vi "SetMethods.vi"(8 "error in (no error)":errorcluster, 10 "Methods":string[](array[string])=["Draw ()", "Scale ()", "Move ()"], 11 "UMLClass in":refnum<class "UMLClass.lvclass">) -> (0 "error out":errorcluster, 3 "UMLClass out":refnum<class "UMLClass.lvclass">)   [LabVIEW 2021, in "Picture2D.lvlib" / "UMLClass.lvclass"]
uses:
  UMLClass.lvclass
  UMLClass.lvclass/UMLClass.ctl
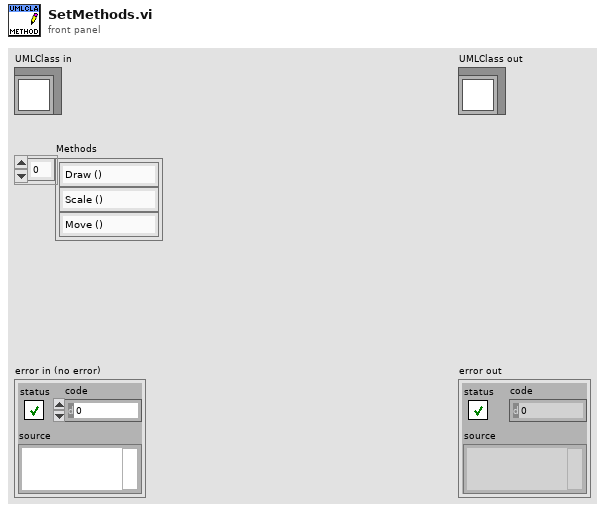
[diagram p1: front panel]
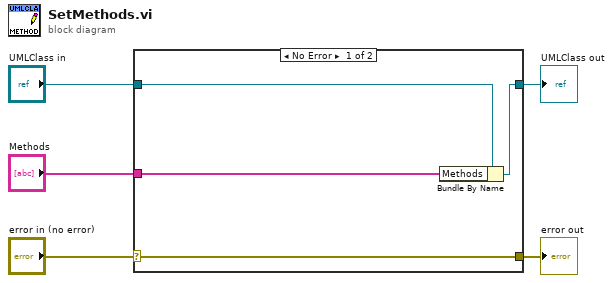
[diagram p0: block diagram]
diagram:
  n1 = case shown="No Error" "error in (no error)" {
    selector: "error in (no error)" -> [w9 w10]
    tunnel: [w9 w10] -> w4
    tunnel: [w7 w11] -> w2
    tunnel: "UMLClass in" -> [w8 w11]
    tunnel: "Methods" -> [w6 _]
    frame No Error {
      n2 = Bundle By Name(cluster=w8, "Methods"=w6) -> (w7:refnum<class "UMLClass.lvclass">)
    }
    frame Error {
    }
  }
  "error out" <- w4
  "UMLClass out" <- w2
